vi "rd_v6_tst_BLK.vi"(1 "ADDRESS 2":i16) -> (0 "Array":u32[](array[numeric]))   [LabVIEW 2015]
doc: "This VI is designed to be used with the UDP Receiver VI. Run the UDP Receiver.vi first.\n\nThe UDP protocol differs from TCP in that there is no error-checking with the packets of information that are sent, and thus no guarantee whatsoever that an intended recipient will actually receive a given piece of data.\n\nUDP does offer the ability to \"broadcast\" data across a network--simply specify an IP Address of all ones (255.255.255.255) to attempt to broadcast information network-wide. Keep in mind that routers and other network hardware will generally refuse to forward the broadcast beyond certain points, so the extent of the broadcast will in practice be limited."
panel:
  out "unsigned 32bit integer":u32
  out "DATA 2":u32
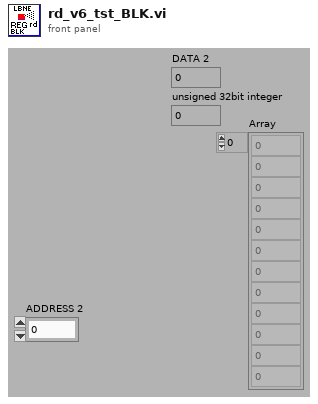
[diagram p1: front panel]
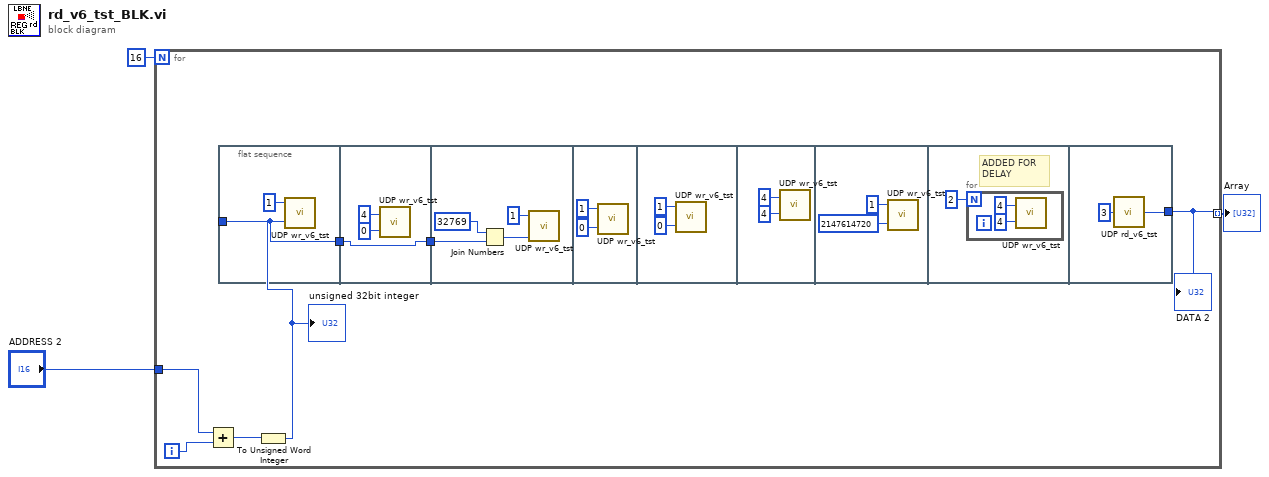
[diagram p0: block diagram]
diagram:
  n1 = for {
    N: 16 -> [_]
    tunnel: "ADDRESS 2" -> [w6]
    tunnel: [w10] -> w1 mode=indexing
    i -> [w7]
    n2 = Add(x=w6, y=w7) -> (x+y=w5:i32)
    n3 = flat-sequence {
      tunnel: w4 -> [w11]
      tunnel: [w11] -> w9
      tunnel: w9 -> [w13]
      tunnel: [w13] -> w8
      tunnel: w8 -> [w17]
      tunnel: [w31] -> w10
      frame #0 {
        n4 = call "UDP wr_v6_tst.vi"("DATA"=w11, "ADDRESS"=u16 1) -> ()  [unwired: 1 out]
      }
      frame #1 {
        n5 = call "UDP wr_v6_tst.vi"("DATA"=u32 0, "ADDRESS"=u16 4) -> ()  [unwired: 1 out]
      }
      frame #2 {
        n6 = Join Numbers(hi=u16 32769, lo=w17) -> ((hi.lo)=w18:u32)
        n7 = call "UDP wr_v6_tst.vi"("DATA"=w18, "ADDRESS"=u16 1) -> ()  [unwired: 1 out]
      }
      frame #3 {
        n8 = call "UDP wr_v6_tst.vi"("DATA"=u32 0, "ADDRESS"=u16 1) -> ()  [unwired: 1 out]
      }
      frame #4 {
        n9 = call "UDP wr_v6_tst.vi"("DATA"=u32 0, "ADDRESS"=u16 1) -> ()  [unwired: 1 out]
      }
      frame #5 {
        n10 = call "UDP wr_v6_tst.vi"("DATA"=u32 4, "ADDRESS"=u16 4) -> ()  [unwired: 1 out]
      }
      frame #6 {
        n11 = call "UDP wr_v6_tst.vi"("DATA"=u32 2147614720, "ADDRESS"=u16 1) -> ()  [unwired: 1 out]
      }
      frame #7 {
        # "ADDED FOR \nDELAY"
        n12 = for {
          N: 2 -> [_]
          n13 = call "UDP wr_v6_tst.vi"("DATA"=u32 4, "ADDRESS"=u16 4) -> ()  [unwired: 1 out]
        }
      }
      frame #8 {
        n14 = call "UDP rd_v6_tst.vi"("ADDRESS 2"=i16 3) -> ("DATA 2"=w31:u32)
      }
    }
    n15 = To Unsigned Word Integer(number=w5) -> (unsigned 16bit integer=w4:u16)
    "unsigned 32bit integer" <- w4
    "DATA 2" <- w10
  }
  "Array" <- w1
